vi "ROI group-Extract selected groups data-Core.vi"(8 "error in":errorcluster) -> (0 "Error out":errorcluster, 1 "X-axis max/min":cluster{"X-axis max":dbl, "X-axis min":dbl}, 2 "Data for ticked Groups":T1)   [LabVIEW 2013]
uses:
  xcontrol/Interface VIs/Interface typedefs/Interface-Data array.ctl
  xcontrol/Interface VIs/Interface typedefs/Interface-Data format definition.ctl
  xcontrol/Typedefs/Xctl-XY data type definition.ctl
  xcontrol/Typedefs/Xctrl-ROI type enum.ctl
  Typedefs/Get-Set-Clear Control.ctl
  Global variables/gl_Functional Imaging-Global variables.vi
  xcontrol/XGrapher.xctl
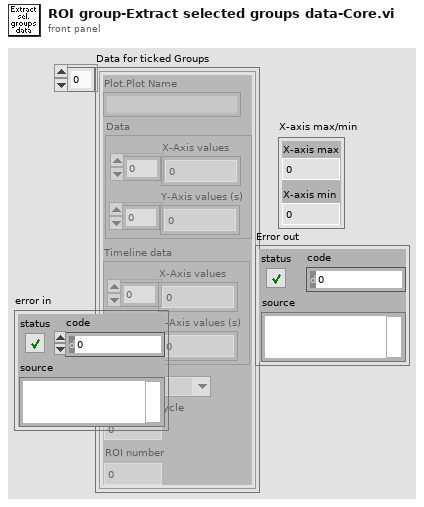
[diagram p1: front panel]
types:
  T1 = typedef "Interface-Data array.ctl" = T2[]
  T2 = typedef "Interface-Data format definition.ctl" = cluster{"Plot.Plot Name":string, "Data":T3, "Timeline data":T3, "Type":T4, "Points per cycle":u16, "ROI number":u16}
  T3 = typedef "XGrapher.xctl/Xctl-XY data type definition.ctl" = cluster{"X-Axis values":sgl[], "Y-Axis values (s)":i32[]}
  T4 = typedef "Xctrl-ROI type enum.ctl" = enum16{"POI", "Mini-scan", "Group"}
  T5 = typedef "Get-Set-Clear Control.ctl" = enum16{"Get", "Set", "Clear"}
  T6 = typedef "Functional Imging UI Refs.ctl" = cluster{"Menu ref":refnum<k9>, "Image control":refnum<vi>, "VI ref":refnum<vi>, "XGrapher":refnum<vi>, "Smoothing":refnum<vi>, "POI Averaging":refnum<vi>, "Normalize":refnum<vi>, "POI data points in each trial":refnum<vi>, "Channel":refnum<vi>, "Experiment data folder path":refnum<vi>, "[ROI vis]":refnum<vi>, "[Groups] visbl":T7, "Group Name":refnum<vi>, "POI index":refnum<vi>, "Trial No.":refnum<vi>, "Intensity Zoom":refnum<vi>, "Trial Cursor Enabled":refnum<vi>, "Number of Trials (ind 1)":refnum<vi>, "Number of Trials (ind 2)":refnum<vi>, "MiniScans Available":refnum<vi>, "POI Available":refnum<vi>, "Defer graph updates":refnum<vi>, "Waveform selector":refnum<vi>, "#of selected POI":refnum<vi>, "#of selected MiniScans":refnum<vi>, "#of selected groups":refnum<vi>, "Max Z-Projection":refnum<vi>, "Z-Plane Selector":refnum<vi>, "Index of miniscan point to visualise":refnum<vi>, "ROI vis. mode":refnum<vi>, "Total # of points":refnum<vi>, "Index of group clicked on":refnum<vi>, "Pane 1":refnum<vi>, "Pane 2":refnum<vi>, "Pane 3":refnum<vi>, "Pane 4":refnum<vi>, "Pane 5":refnum<vi>, "Pane 6":refnum<vi>, "Deselect all ROI":refnum<vi>, "Deselect all groups":refnum<vi>}
  T7 = typedef "Groups array referecne.ctl" = refnum<vi>
  T8 = typedef "Group sel cluster.ctl" = cluster{"Group number":string, "Group Name":string, "Visibility":bool, "Highlight":bool}
  T9 = typedef "ROI group info cluster.ctl" = cluster{"Group name":string, "# ROI in group":i32, "ROI numbers in group":i32[], "Group region specifier cluster":T10}
  T10 = typedef "ROI Descriptor" = cluster{"Global Rectangle":i32[], "Contours":cluster{"ID":enum32{"External", "Internal"}, "Type":u32, "Coordinates":i32[]}[]}
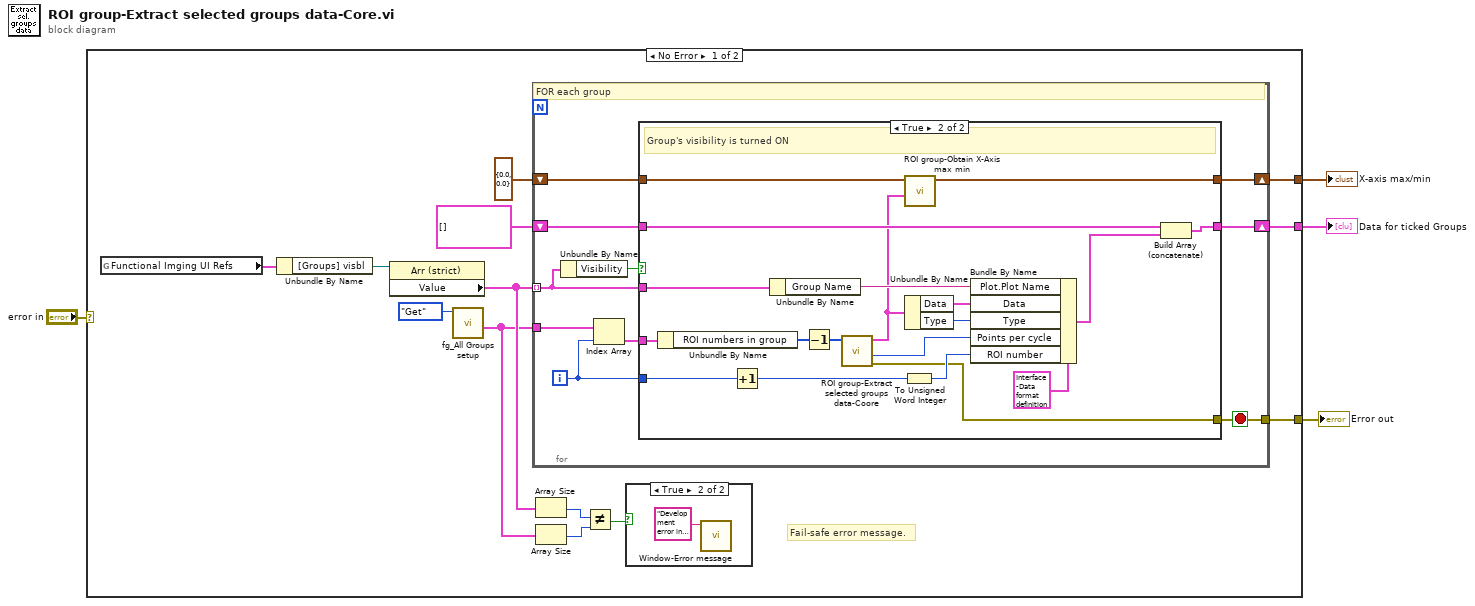
[diagram p0: block diagram]
diagram:
  n1 = case shown="No Error" "error in" {
    selector: "error in" -> [_ w50]
    tunnel: [w15 _] -> w4
    tunnel: [w6 _] -> w3
    tunnel: [w5 w50] -> w2
    frame No Error {
      # "Fail-safe error message."
      n2 = global read "gl_Functional Imaging-Global variables.vi" "Functional Imging UI Refs"() -> (w13:T6)
      n3 = Unbundle By Name(w13) -> ("[Groups] visbl"=w16:T7)
      n4 = property on="Property Node" class="Arr (strict)"(reference=w16) -> ("Value"=w12:T8[])  [unwired: 1 in, 2 out]
      n5 = call "fg_All Groups setup.vi"("Function"=Get-Set-Clear_Control."Get") -> ("Groups setup out"=w11:T9[])  [unwired: 9 in, 1 out]
      n6 = for {
        tunnel: w12 -> [w25] mode=indexing
        tunnel: w11 -> [w24]
        shift-right: [w26] -> w15
        shift-left: T1 [] ("Data for ticked Groups") -> [w27]
        shift-right: [w21] -> w6
        shift-left: cluster{"Max":dbl, "Min":dbl} {"Max"=0.0, "Min"=0.0} -> [w20]
        tunnel: [w19] -> w5
        i -> [w22]
        stop <- w19 stop-if-true
        # "FOR each group"
        n7 = Unbundle By Name(w25) -> ("Visibility"=w28:bool)
        n8 = Index Array(array=w24, index=w22) -> (element=w23:T9)
        n9 = case shown="True" w28 {
          tunnel: w23 -> [_ w49]
          tunnel: [w30 w44] -> w26
          tunnel: w27 -> [w30 w45]
          tunnel: w25 -> [_ w43]
          tunnel: w22 -> [_ w41]
          tunnel: [w29 w34] -> w21
          tunnel: w20 -> [w29 w33]
          tunnel: [_ w31] -> w19
          frame False {
            # "Group's visibility is OFF"
          }
          frame True {
            # "Group's visibility is turned ON"
            n10 = Unbundle By Name(w49) -> ("ROI numbers in group"=w42:i32[])
            n11 = Increment(x=w41) -> (x+1=w40:i32)
            n12 = Unbundle By Name(w43) -> ("Group Name"=w48:string)
            n13 = Decrement(x=w42) -> (x-1=w37:i32[])
            n14 = call "ROI group-Extract selected groups data-Coore.vi"("Indexes of ROI in group"=w37) -> ("error IO"=w31:errorcluster, "Points per cycle"=w38:u16, "ROI group data"=w32:T2)  [unwired: 8 in]
            n15 = To Unsigned Word Integer(number=w40) -> (unsigned 16bit integer=w39:u16)
            n16 = call "ROI group-Obtain X-Axis max min.vi"("ROI group data"=w32, "Max min-shift in"=w33) -> ("Max min out"=w34:cluster{dbl, dbl})  [unwired: 9 in]
            n17 = Unbundle By Name(w32) -> ("Data"=w36:T3, "Type"=w35:T4)
            n18 = Bundle By Name(cluster=T2 {"Plot.Plot Name"="", "Data"={"X-Axis values"=[], "Y-Axis values (s)"=[]}, "Timeline data"={"X-Axis values"=[], "Y-Axis values (s)"=[]}, "Type"=enum."POI", "Points per cycle"=0, "ROI number"=0}, "Plot.Plot Name"=w48, "Data"=w36, "Type"=w35, "Points per cycle"=w38, "ROI number"=w39) -> (w46:T2)
            n19 = Build Array (concatenate)(w45, w46) -> (w44:T1)
          }
        }
      }
      n20 = Array Size(array=w12) -> (size(s)=w10:i32)
      n21 = Array Size(array=w11) -> (size(s)=w9:i32)
      n22 = Not Equal?(x=w10, y=w9) -> (x != y?=w8:bool)
      n23 = case shown="True" w8 {
        frame False {
        }
        frame True {
          n24 = call "Window-Error message.vi"("Message"="Development error in the \"ROI group-Extract selected groups data-Core.vi\"\nArray mismatch.") -> ()  [unwired: 10 in, 1 out]
        }
      }
    }
    frame Error {
    }
  }
  "Data for ticked Groups" <- w4
  "X-axis max/min" <- w3
  "Error out" <- w2
